vi "Auton File Control.vi"(9 "D-Pad":T2, 10 "Button Cluster":T1) -> ()   [LabVIEW 2016]
uses:
  Common Code/Gamepads/D-Pad.ctl
  Common Code/Gamepads/Button Cluster.ctl
  Common Code/Utilities/Change Detect Double.vi
  Common Code/Utilities/Change Detect Boolean.vi
  Common Code/Utilities/Change Detect Int.vi
  Robot Global Data.vi
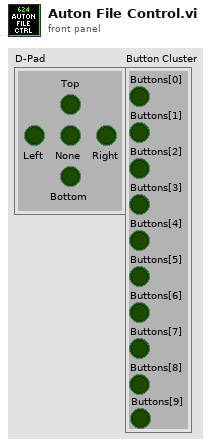
[diagram p1: front panel]
types:
  T1 = typedef "Button Cluster.ctl" = cluster{"Buttons[0]":bool, "Buttons[1]":bool, "Buttons[2]":bool, "Buttons[3]":bool, "Buttons[4]":bool, "Buttons[5]":bool, "Buttons[6]":bool, "Buttons[7]":bool, "Buttons[8]":bool, "Buttons[9]":bool}
  T2 = typedef "D-Pad.ctl" = cluster{"Top":bool, "Bottom":bool, "None":bool, "Right":bool, "Left":bool}
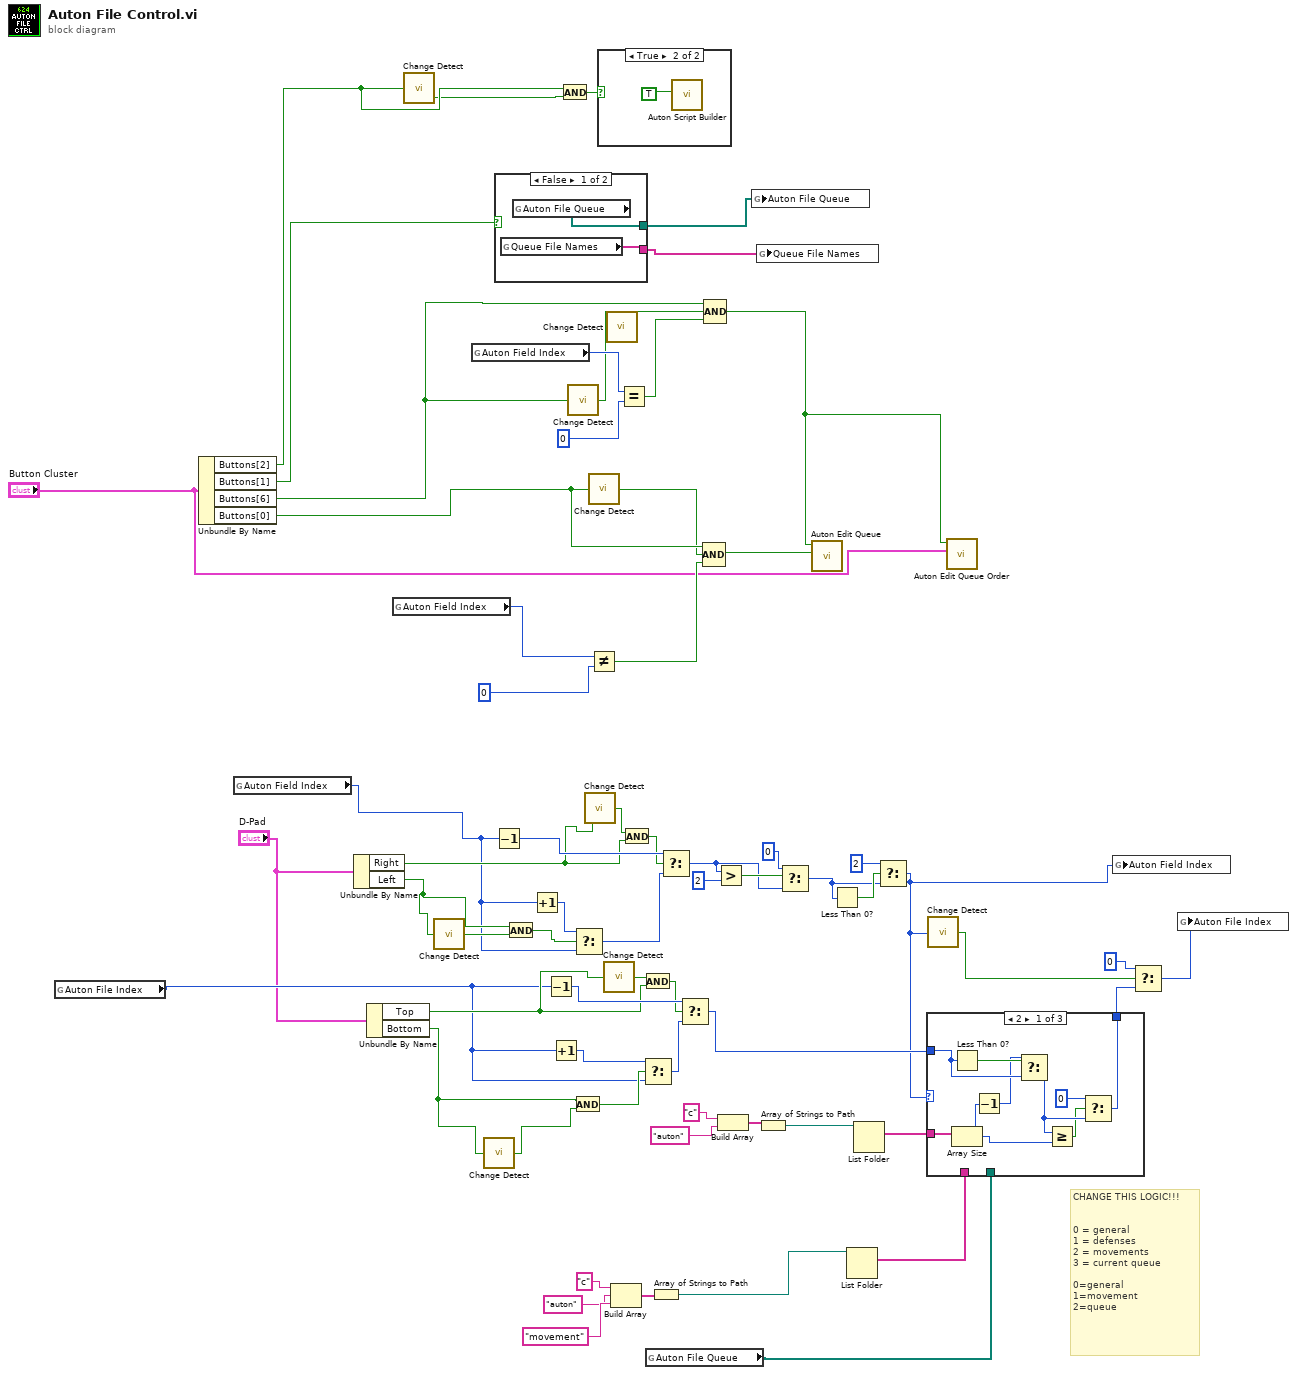
[diagram p0: block diagram]
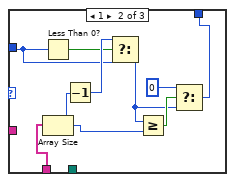
[diagram p2: hidden frame]
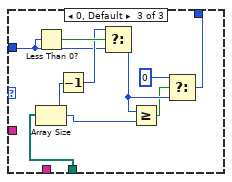
[diagram p3: hidden frame]
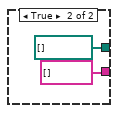
[diagram p5: hidden frame]
diagram:
  # "CHANGE THIS LOGIC!!! \n\n\n0 = general \n1 = defenses \n2 = movements\n3 = current queue\n\n0=general \n1=movement \n2=queue"
  n1 = global read "Robot Global Data.vi" "Auton File Index"() -> (w3:i32)
  n2 = Unbundle By Name("Button Cluster") -> ("Buttons[2]"=w48:bool, "Buttons[1]"=w49:bool, "Buttons[6]"=w54:bool, "Buttons[0]"=w61:bool)
  n3 = global read "Robot Global Data.vi" "Auton Field Index"() -> (w2:i32)
  n4 = Unbundle By Name("D-Pad") -> ("Right"=w9:bool, "Left"=w15:bool)
  n5 = Unbundle By Name("D-Pad") -> ("Top"=w12:bool, "Bottom"=w11:bool)
  n6 = global read "Robot Global Data.vi" "Auton Field Index"() -> (w64:i32)
  n7 = call-poly "Change Detect.vi"("In"=w48) -> ("Changed?"=w47:bool)
  n8 = call-poly "Change Detect.vi"("In"=w15) -> ("Changed?"=w14:bool)
  n9 = global read "Robot Global Data.vi" "Auton Field Index"() -> (w59:i32)
  n10 = call-poly "Change Detect.vi"("In"=w11) -> ("Changed?"=w10:bool)
  n11 = Decrement(x=w2) -> (x-1=w46:i32)
  n12 = case shown="False" w49 {
    tunnel: [w67 path[] [] ("Auton File Queue")] -> w51
    tunnel: [w66 string[] [] ("Queue File Names")] -> w50
    frame False {
      n13 = global read "Robot Global Data.vi" "Queue File Names"() -> (w66:string[])
      n14 = global read "Robot Global Data.vi" "Auton File Queue"() -> (w67:path[])
    }
    frame True {
    }
  }
  n15 = And(x=w15, y=w14) -> (x .and. y?=w18:bool)
  n16 = Increment(x=w2) -> (x+1=w45:i32)
  n17 = Decrement(x=w3) -> (x-1=w34:i32)
  n18 = Increment(x=w3) -> (x+1=w35:i32)
  n19 = And(x=w48, y=w47) -> (x .and. y?=w52:bool)
  n20 = call-poly "Change Detect.vi"("In"=w54) -> ("Changed?"=w53:bool)
  n21 = And(x=w11, y=w10) -> (x .and. y?=w16:bool)
  n22 = Select(t=w45, s=w18, f=w2) -> (s? t:f=w44:i32)
  n23 = call-poly "Change Detect.vi"("In"=w9) -> ("Changed?"=w8:bool)
  n24 = call-poly "Change Detect.vi"("In"=w61) -> ("Changed?"=w60:bool)
  n25 = Not Equal?(x=w64, y=0 ("Auton Field Index")) -> (x != y?=w63:bool)
  n26 = case shown="True" w52 {
    frame False {
    }
    frame True {
      n27 = call "Auton Script Builder.vi"("Export?"=TRUE) -> ()  [unwired: 10 in, 1 out]
    }
  }
  n28 = call-poly "Change Detect.vi"("In"=w12) -> ("Changed?"=w13:bool)
  n29 = call-poly "Change Detect.vi"() -> ()  [unwired: 1 in, 1 out]
  n30 = Build Array("c", "auton", "movement" ("element")) -> (w27:string[])
  n31 = Equal?(x=w59, y=0 ("Auton Field Index")) -> (x = y?=w57:bool)
  n32 = And(x=w8, y=w9) -> (x .and. y?=w19:bool)
  n33 = And(x=w13, y=w12) -> (x .and. y?=w17:bool)
  n34 = Select(t=w35, s=w16, f=w3) -> (s? t:f=w36:i32)
  n35 = global read "Robot Global Data.vi" "Auton File Queue"() -> (w6:path[])
  n36 = Array of Strings to Path(0:w27) -> (2:w25:path)  [unwired: 1 in]
  n37 = Select(t=w46, s=w19, f=w44) -> (s? t:f=w41:i32)
  n38 = Select(t=w34, s=w17, f=w36) -> (s? t:f=w33:i32)
  n39 = Compound Arithmetic op=AND(w61, w60, w63) -> (w62:bool)
  n40 = Compound Arithmetic op=AND(w54, w53, w57) -> (w56:bool)
  n41 = Greater?(x=w41, y=2) -> (0:w42:bool)
  n42 = Build Array("c", "auton") -> (w22:string[])
  n43 = global write "Robot Global Data.vi" "Auton File Queue"(w51) -> ()
  n44 = global write "Robot Global Data.vi" "Queue File Names"(w50) -> ()
  n45 = Array of Strings to Path(0:w22) -> (2:w20:path)  [unwired: 1 in]
  n46 = Select(t=0, s=w42, f=w41) -> (s? t:f=w38:i32)
  n47 = call "Auton Edit Queue.vi"("Add?"=w62, "Delete?"=w56) -> ()  [unwired: 10 in]
  n48 = Less Than 0?(x=w38) -> (x < 0?=w39:bool)
  n49 = List Folder(path=w25) -> (filenames=w31:string[])  [unwired: 3 in, 3 out]
  n50 = List Folder(path=w20) -> (filenames=w32:string[])  [unwired: 3 in, 3 out]
  n51 = Select(t=2, s=w39, f=w38) -> (s? t:f=w4:i32)
  n52 = case shown="2" w4 {
    tunnel: w33 -> [w77 w81 w90]
    tunnel: w32 -> [w79 _ _]
    tunnel: w31 -> [_ w82 _]
    tunnel: w6 -> [_ _ w89]
    tunnel: [w71 w80 w91] -> w30
    frame 2 {
      n53 = Less Than 0?(x=w77) -> (x < 0?=w78:bool)
      n54 = Array Size(array=w79) -> (size(s)=w74:i32)
      n55 = Decrement(x=w74) -> (x-1=w76:i32)
      n56 = Select(t=w76, s=w78, f=w77) -> (s? t:f=w75:i32)
      n57 = Greater Or Equal?(x=w75, y=w74) -> (x >= y?=w73:bool)
      n58 = Select(t=0, s=w73, f=w75) -> (s? t:f=w71:i32)
    }
    frame 1 {
      n59 = Less Than 0?(x=w81) -> (x < 0?=w83:bool)
      n60 = Array Size(array=w82) -> (size(s)=w86:i32)
      n61 = Decrement(x=w86) -> (x-1=w84:i32)
      n62 = Select(t=w84, s=w83, f=w81) -> (s? t:f=w85:i32)
      n63 = Greater Or Equal?(x=w85, y=w86) -> (x >= y?=w87:bool)
      n64 = Select(t=0, s=w87, f=w85) -> (s? t:f=w80:i32)
    }
    frame 0, Default {
      n65 = Less Than 0?(x=w90) -> (x < 0?=w97:bool)
      n66 = Array Size(array=w89) -> (size(s)=w94:i32)
      n67 = Decrement(x=w94) -> (x-1=w96:i32)
      n68 = Select(t=w96, s=w97, f=w90) -> (s? t:f=w95:i32)
      n69 = Greater Or Equal?(x=w95, y=w94) -> (x >= y?=w93:bool)
      n70 = Select(t=0, s=w93, f=w95) -> (s? t:f=w91:i32)
    }
  }
  n71 = call-poly "Change Detect.vi"("In"=w4) -> ("Changed?"=w7:bool)
  n72 = call "Auton Edit Queue Order.vi"("Button Cluster"="Button Cluster", "Boolean"=w56) -> ()  [unwired: 10 in]
  n73 = global write "Robot Global Data.vi" "Auton Field Index"(w4) -> ()
  n74 = Select(t=0, s=w7, f=w30) -> (s? t:f=w5:i32)
  n75 = global write "Robot Global Data.vi" "Auton File Index"(w5) -> ()
